vi "packaging-rpm.vi"(3 "Thermometer in":dbl(slide) scale=0.0..200.0, 4 "state in":T1, 5 "speed in":i32(listbox)) -> (0 "Thermometer out":dbl(slide) scale=0.0..200.0, 2 "rpm out":dbl(knob) scale=0.0..10.0)   [LabVIEW 2026]
uses:
  Packaging-machine-state-machine.ctl
  <vilib>/numeric/Random Number (Range) DBL.vi
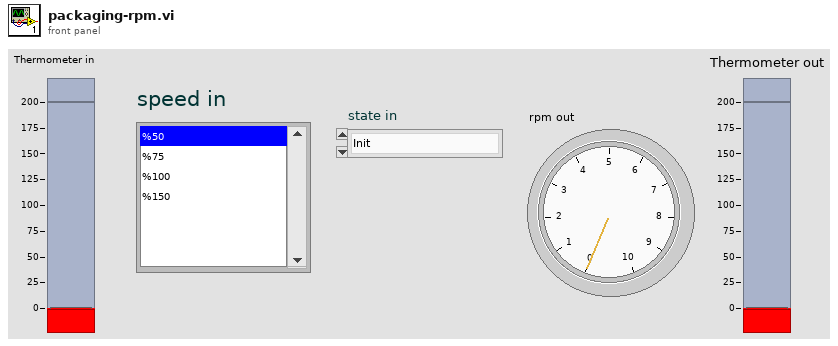
[diagram p1: front panel]
types:
  T1 = typedef "Packaging-machine-state-machine.ctl" = enum16{"Init", "Ready", "Running", "Emergency"}
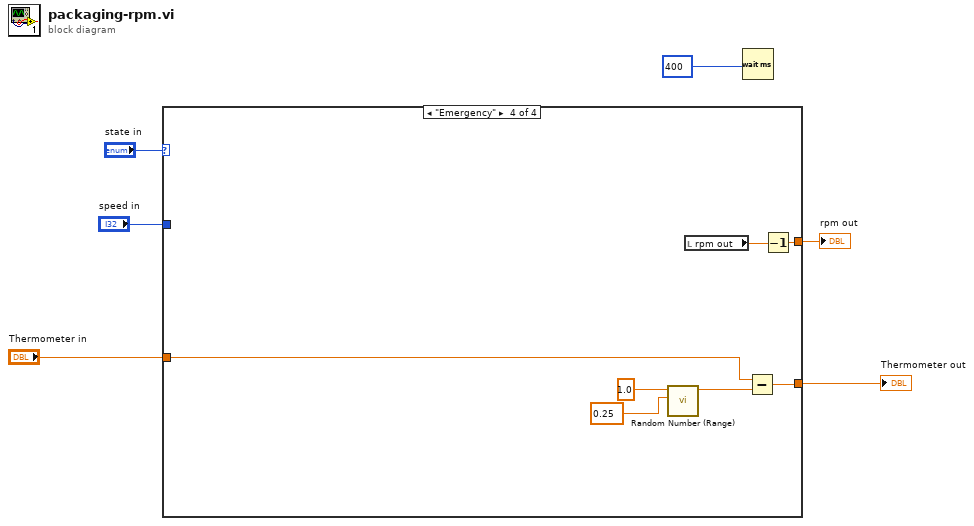
[diagram p0: block diagram]
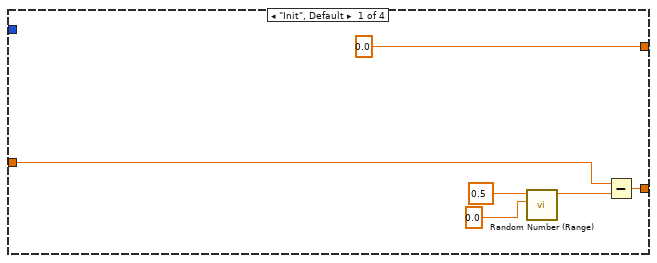
[diagram p2: hidden frame]
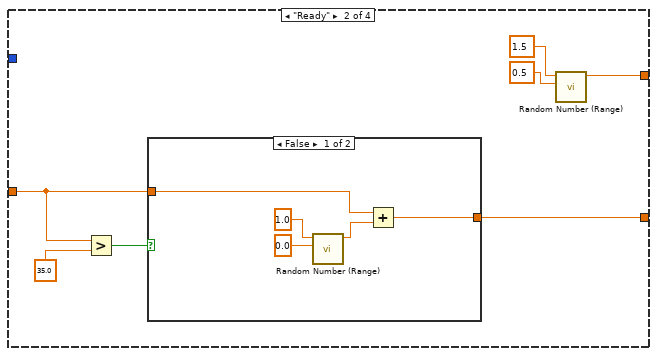
[diagram p3: hidden frame]
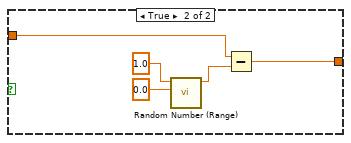
[diagram p4: hidden frame]
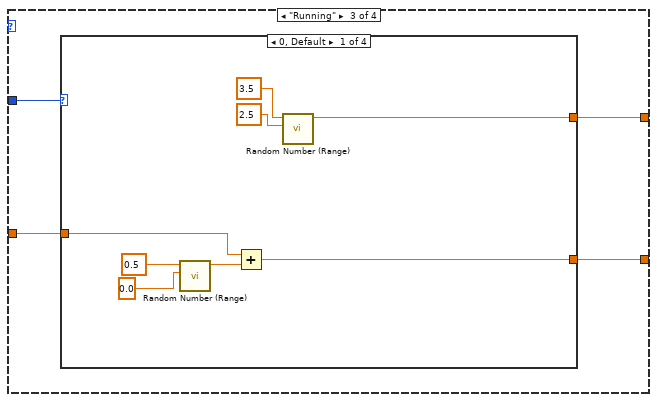
[diagram p5: hidden frame]
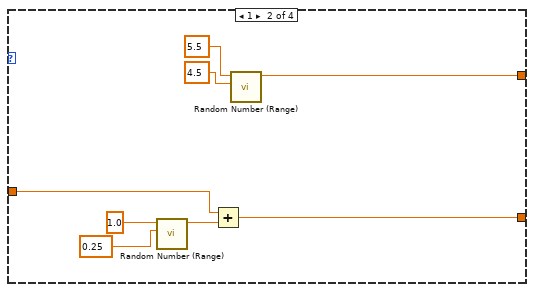
[diagram p6: hidden frame]
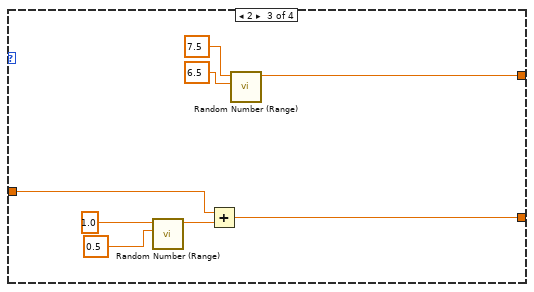
[diagram p7: hidden frame]
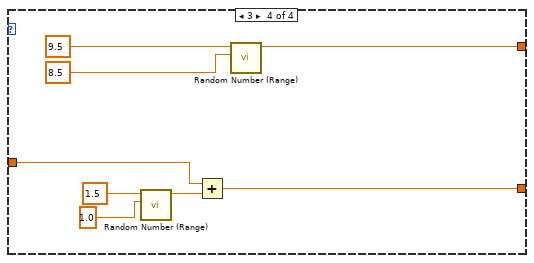
[diagram p8: hidden frame]
diagram:
  n1 = case shown="\"Emergency\"" "state in" {
    tunnel: [0.0 ("number") w17 w32 w72] -> w5
    tunnel: "speed in" -> [_ _ w33 _]
    tunnel: "Thermometer in" -> [w7 w14 w31 w66]
    tunnel: [w9 w13 w30 w67] -> w2
    frame "Init", Default {
      n2 = call-poly <vilib>:"Random Number (Range).vi"("lower bound (0)"=0.0, "upper bound (100)"=0.5) -> ("number"=w8:dbl)  [unwired: 9 in]
      n3 = Subtract(x=w7, y=w8) -> (x-y=w9:dbl)
    }
    frame "Ready" {
      n4 = Greater?(x=w14, y=35.0) -> (0:w16:bool)
      n5 = case shown="False" w16 {
        tunnel: w14 -> [w20 w27]
        tunnel: [w21 w25] -> w13
        frame False {
          n6 = call-poly <vilib>:"Random Number (Range).vi"("lower bound (0)"=0.0, "upper bound (100)"=1.0) -> ("number"=w22:dbl)  [unwired: 9 in]
          n7 = Add(x=w20, y=w22) -> (x+y=w21:dbl)
        }
        frame True {
          n8 = call-poly <vilib>:"Random Number (Range).vi"("lower bound (0)"=0.0, "upper bound (100)"=1.0) -> ("number"=w26:dbl)  [unwired: 9 in]
          n9 = Subtract(x=w27, y=w26) -> (x-y=w25:dbl)
        }
      }
      n10 = call-poly <vilib>:"Random Number (Range).vi"("lower bound (0)"=0.5, "upper bound (100)"=1.5) -> ("number"=w17:dbl)  [unwired: 9 in]
    }
    frame "Running" {
      n11 = case shown="0, Default" w33 {
        tunnel: [w39 w47 w55 w63] -> w32
        tunnel: w31 -> [w35 w43 w50 w59]
        tunnel: [w34 w42 w51 w58] -> w30
        frame 0, Default {
          n12 = call-poly <vilib>:"Random Number (Range).vi"("lower bound (0)"=0.0, "upper bound (100)"=0.5) -> ("number"=w36:dbl)  [unwired: 9 in]
          n13 = Add(x=w35, y=w36) -> (x+y=w34:dbl)
          n14 = call-poly <vilib>:"Random Number (Range).vi"("lower bound (0)"=2.5, "upper bound (100)"=3.5) -> ("number"=w39:dbl)  [unwired: 9 in]
        }
        frame 1 {
          n15 = call-poly <vilib>:"Random Number (Range).vi"("lower bound (0)"=0.25, "upper bound (100)"=1.0) -> ("number"=w44:dbl)  [unwired: 9 in]
          n16 = Add(x=w43, y=w44) -> (x+y=w42:dbl)
          n17 = call-poly <vilib>:"Random Number (Range).vi"("lower bound (0)"=4.5, "upper bound (100)"=5.5) -> ("number"=w47:dbl)  [unwired: 9 in]
        }
        frame 2 {
          n18 = call-poly <vilib>:"Random Number (Range).vi"("lower bound (0)"=0.5, "upper bound (100)"=1.0) -> ("number"=w54:dbl)  [unwired: 9 in]
          n19 = Add(x=w50, y=w54) -> (x+y=w51:dbl)
          n20 = call-poly <vilib>:"Random Number (Range).vi"("lower bound (0)"=6.5, "upper bound (100)"=7.5) -> ("number"=w55:dbl)  [unwired: 9 in]
        }
        frame 3 {
          n21 = call-poly <vilib>:"Random Number (Range).vi"("lower bound (0)"=1.0, "upper bound (100)"=1.5) -> ("number"=w60:dbl)  [unwired: 9 in]
          n22 = Add(x=w59, y=w60) -> (x+y=w58:dbl)
          n23 = call-poly <vilib>:"Random Number (Range).vi"("lower bound (0)"=8.5, "upper bound (100)"=9.5) -> ("number"=w63:dbl)  [unwired: 9 in]
        }
      }
    }
    frame "Emergency" {
      n24 = call-poly <vilib>:"Random Number (Range).vi"("lower bound (0)"=0.25, "upper bound (100)"=1.0) -> ("number"=w70:dbl)  [unwired: 9 in]
      n25 = local read "rpm out"() -> (w71:dbl)
      n26 = Subtract(x=w66, y=w70) -> (x-y=w67:dbl)
      n27 = Decrement(x=w71) -> (x-1=w72:dbl)
    }
  }
  "rpm out" <- w5
  "Thermometer out" <- w2
  n28 = Wait (ms)(milliseconds to wait=u32 400) -> ()  [unwired: 1 out]
